vi "Launcher.vi"() -> ()   [LabVIEW 2014]
uses:
  XShelxtlLauncherDll.dll
panel:
  in  "Target file":path
  in  "Parameter File 3":path
  in  "Parameter File 2":path
  in  "Parameter File 1":path
  in  "Shelxt.exe Path":path
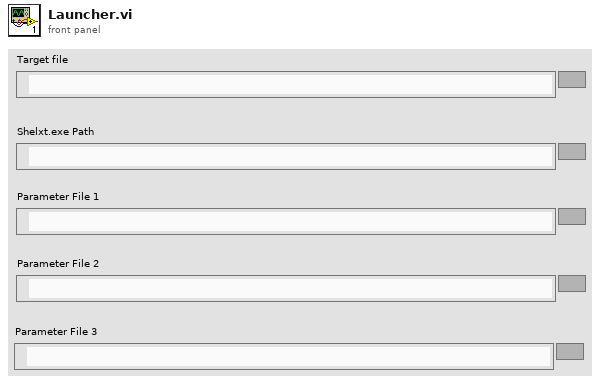
[diagram p1: front panel]
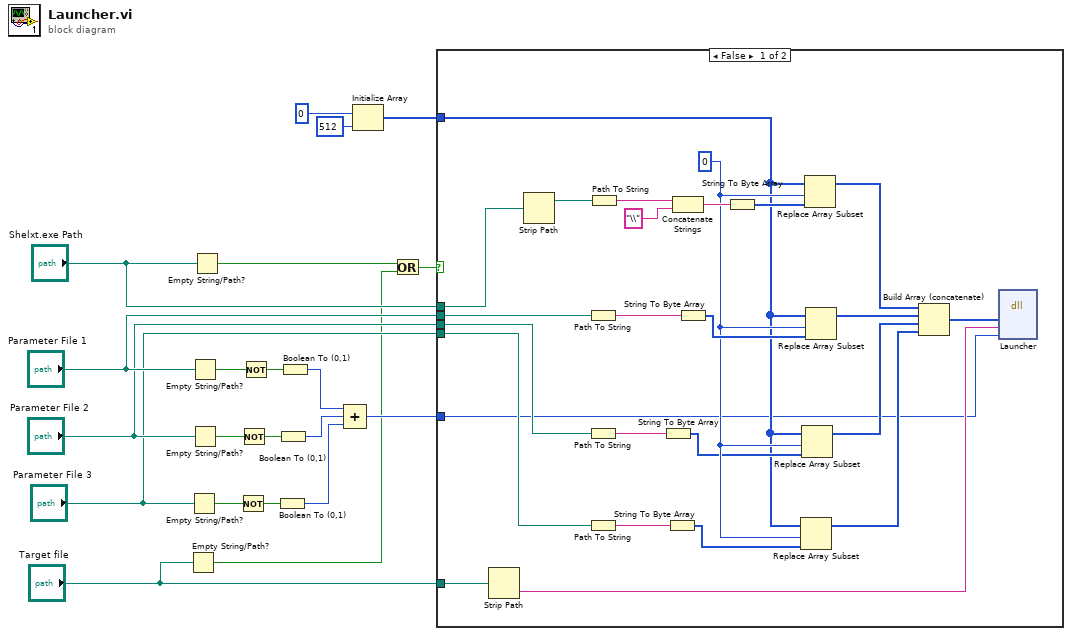
[diagram p0: block diagram]
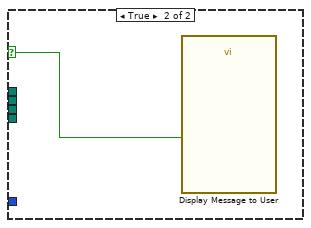
[diagram p2: hidden frame]
diagram:
  n1 = Empty String/Path?(string/path="Target file") -> (empty?=w5:bool)
  n2 = Empty String/Path?(string/path="Parameter File 3") -> (empty?=w16:bool)
  n3 = Empty String/Path?(string/path="Parameter File 1") -> (empty?=w21:bool)
  n4 = Empty String/Path?(string/path="Parameter File 2") -> (empty?=w18:bool)
  n5 = Empty String/Path?(string/path="Shelxt.exe Path") -> (empty?=w4:bool)
  n6 = Not(x=w16) -> (.not. x?=w17:bool)
  n7 = Not(x=w18) -> (.not. x?=w19:bool)
  n8 = Not(x=w21) -> (.not. x?=w20:bool)
  n9 = Boolean To (0,1)(Boolean=w17) -> (0, 1=w13:i16)
  n10 = Boolean To (0,1)(Boolean=w19) -> (0, 1=w14:i16)
  n11 = Boolean To (0,1)(Boolean=w20) -> (0, 1=w15:i16)
  n12 = Compound Arithmetic op=ADD(w15, w14, w13) -> (w8:i16)
  n13 = Initialize Array(u8 0, 512 ("dimension size")) -> (w1:u8[])
  n14 = Or(x=w4, y=w5) -> (x .or. y?=w6:bool)
  n15 = case shown="False" w6 {
    selector: w6 -> [_ w47]
    tunnel: "Shelxt.exe Path" -> [w46 _]
    tunnel: "Parameter File 1" -> [w44 _]
    tunnel: "Parameter File 2" -> [w43 _]
    tunnel: "Parameter File 3" -> [w42 _]
    tunnel: w8 -> [w22 _]
    tunnel: "Target file" -> [w41 _]
    tunnel: w1 -> [w30 _]
    frame False {
      w32 = 0 ("index")
      n16 = Strip Path(path=w41) -> (name=w23:string)  [unwired: 1 out]
      n17 = Strip Path(path=w46) -> (stripped path=w45:path)  [unwired: 1 out]
      n18 = Path To String(path=w44) -> (string=w27:string)
      n19 = Path To String(path=w43) -> (string=w26:string)
      n20 = Path To String(path=w42) -> (string=w25:string)
      n21 = Path To String(path=w45) -> (string=w28:string)
      n22 = String To Byte Array(string=w26) -> (unsigned byte array=w31:u8[])
      n23 = String To Byte Array(string=w25) -> (unsigned byte array=w29:u8[])
      n24 = Concatenate Strings(w28, "\\") -> (w39:string)
      n25 = String To Byte Array(string=w27) -> (unsigned byte array=w33:u8[])
      n26 = String To Byte Array(string=w39) -> (unsigned byte array=w34:u8[])
      n27 = Replace Array Subset(array=w30, new element=w29, index=w32) -> (w35:u8[])
      n28 = Replace Array Subset(array=w30, new element=w31, index=w32) -> (w36:u8[])
      n29 = Replace Array Subset(array=w30, new element=w34, index=w32) -> (w38:u8[])
      n30 = Replace Array Subset(array=w30, new element=w33, index=w32) -> (w37:u8[])
      n31 = Build Array (concatenate)(w38, w37, w36, w35) -> (w24:u8[])
      n32 = dll-call lib="C:/Users/DrippySummer/Documents/LabVIEW Data/SavaData/XShelxtlLauncher/XShelxtlLauncherDll.dll" fn="Launcher"("strList"=w24, "targetFile"=w23, "paraNum"=w22) -> ()  [unwired: 7 in, 2 out]
    }
    frame True {
      n33 = call "Display Message to User"("Enable"=w47) -> ()  [unwired: 9 in, 2 out]
    }
  }
